vi "Determine Action.vi"(8 "Updated View":i32[](array[numeric]) caption="Updated View (-1 team, 0 empty, 1 enemy)", 9 "Column":i32, 10 "Row":i32, 11 "Great Wall in":refnum<class "Great Wall.lvclass">) -> (1 "Direction":T1, 2 "Action":T2, 3 "Great Wall out":refnum<class "Great Wall.lvclass">)   [LabVIEW 2015, in "Great Wall.lvclass"]
uses:
  Great Wall.lvclass
  DS Square Library/DS Square.lvlib
  Type Defs/Action Enum.ctl
  Type Defs/SB Type Defs.lvlib
  Type Defs/Direction Enum.ctl
  Square/Square.lvclass
  Wall State Enum.ctl
panel:
  # "NW\nN\nNE\nE\nSE\nS\nSW\nW"
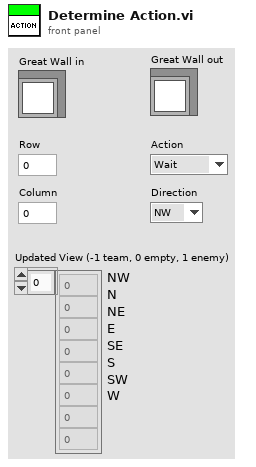
[diagram p1: front panel]
types:
  T1 = typedef "SB Type Defs.lvlib/Direction Enum.ctl" = enum16{"NW", "N", "NE", "E", "SE", "S", "SW", "W"}
  T2 = typedef "SB Type Defs.lvlib/Action Enum.ctl" = enum16{"Wait", "Move", "Attack", "Replicate"}
  T3 = typedef "Great Wall.lvclass/Wall State Enum.ctl" = enum16{"Under Construction", "Hold", "Advance 1", "Advance 2", "Retreat"}
  T4 = typedef "Great Wall.lvclass/Private Data.ctl" = cluster{"wall 1":T5, "wall 2":T5, "start row":i32, "start col":i32, "state update round":i32}
  T5 = typedef "Great Wall.lvclass/Wall State.ctl" = cluster{"state":T3, "direction":T1, "index":i32}
  T6 = typedef "Great Wall.lvclass/Square Mode.ctl" = enum16{"Replicator", "Guard", "Wall"}
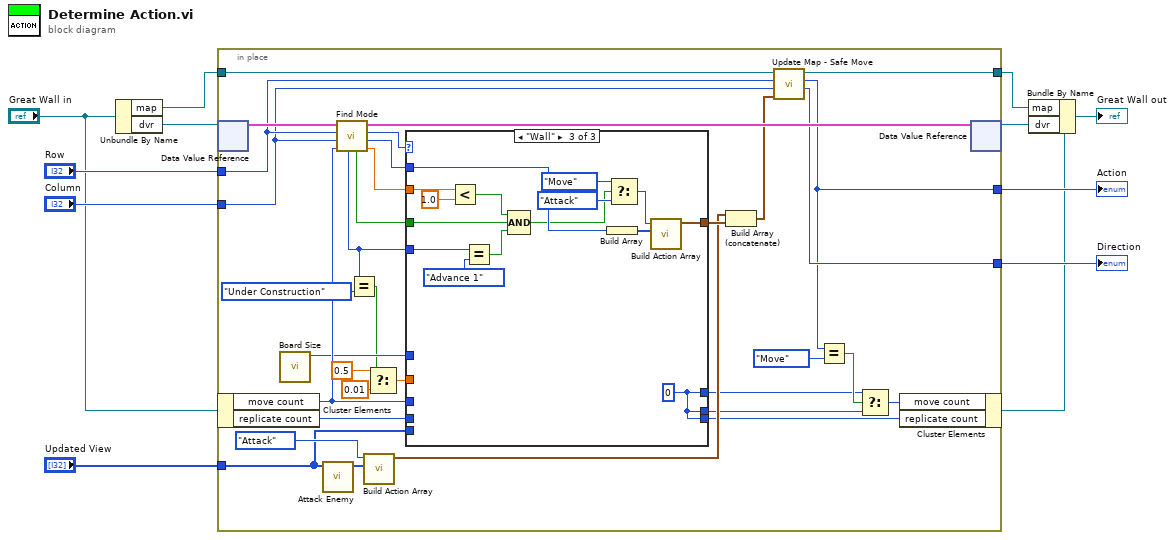
[diagram p0: block diagram]
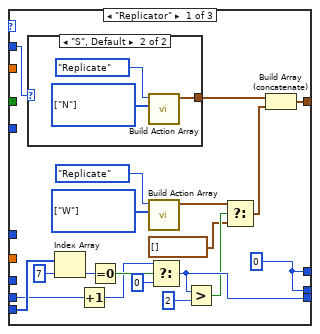
[diagram p2: hidden frame]
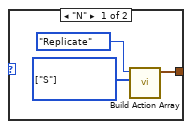
[diagram p3: hidden frame]
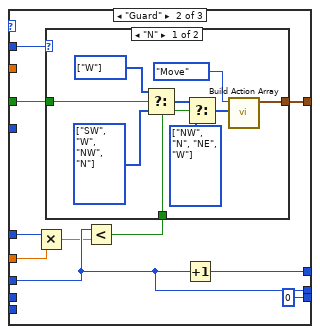
[diagram p4: hidden frame]
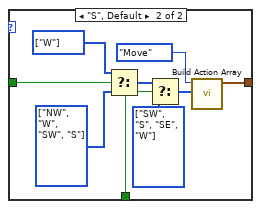
[diagram p5: hidden frame]
diagram:
  n1 = Unbundle By Name("Great Wall in") -> ("map"=w7:refnum<data-value>, "dvr"=w12:refnum<data-value>)
  n2 = in-place {
    in-place-border: "Row" -> [w34]
    in-place-border: "Column" -> [w33]
    in-place-border: w7 -> [w44]
    in-place-border: "Updated View" -> [w21]
    in-place-border: [w43] -> w5
    in-place-border: [w31] -> w4
    in-place-border: [w32] -> w3
    n3 = in-place-dvr #1(w12) -> (w45:T4)  [unwired: 1 out]
    n4 = in-place-cluster #2("Great Wall in") -> ("move count"=w25:i32, "replicate count"=w24:i32)
    n5 = call "Board Size.vi"() -> ("Board Size"=w20:i32)  [unwired: 11 in]
    n6 = call "Attack Enemy.vi"("View in"=w21) -> ("all enemies"=w22:T1[])  [unwired: 8 in, 2 out]
    n7 = call "Find Mode.vi"("move count"=w25, "Column"=w33, "Row"=w34, "private data in"=w45) -> ("distance"=w13:dbl, "nearest wall"=w39:T1, "mode"=w41:T6, "private data out"=w42:T4, "even?"=w35:bool, "wall state"=w19:T3)  [unwired: 2 in]
    n8 = Equal?(x=w19, y=Wall_State_Enum."Under Construction") -> (x = y?=w17:bool)
    n9 = call "Build Action Array.vi"("directions"=w22, "Action"=Action_Enum."Attack") -> ("actions"=w37:cluster{"Action":T2, "Direction":T1}[])  [unwired: 9 in]
    n10 = Select(t=0.5, s=w17, f=0.01) -> (s? t:f=w16:dbl)
    n11 = case shown="\"Wall\"" w41 {
      tunnel: w39 -> [w64 w80 w112]
      tunnel: [w60 w79 w113] -> w38
      tunnel: w25 -> [_ w75 _]
      tunnel: [w63 w78 w105] -> w28
      tunnel: w35 -> [_ w77 w104]
      tunnel: [w63 w75 w105] -> w26
      tunnel: w19 -> [_ _ w110]
      tunnel: w24 -> [w53 _ _]
      tunnel: [w50 0 ("replicate count") w105] -> w23
      tunnel: w21 -> [w57 _ _]
      tunnel: w20 -> [_ w72 _]
      tunnel: w16 -> [_ w71 _]
      tunnel: w13 -> [_ _ w101]
      frame "Replicator" {
        w61 = T1[] [enum."W"] items=["NW", "N", "NE", "E", "SE", "S", "SW", "W"] ("all enemies")
        w63 = 0
        n12 = case shown="\"S\", Default" w64 {
          tunnel: [w65 w68] -> w59
          frame "N" {
            w67 = T1[] [enum."S"] items=["NW", "N", "NE", "E", "SE", "S", "SW", "W"] ("all enemies")
            n13 = call "Build Action Array.vi"("directions"=w67, "Action"=Action_Enum."Replicate") -> ("actions"=w65:cluster{"Action":T2, "Direction":T1}[])  [unwired: 9 in]
          }
          frame "S", Default {
            w70 = T1[] [enum."N"] items=["NW", "N", "NE", "E", "SE", "S", "SW", "W"] ("all enemies")
            n14 = call "Build Action Array.vi"("directions"=w70, "Action"=Action_Enum."Replicate") -> ("actions"=w68:cluster{"Action":T2, "Direction":T1}[])  [unwired: 9 in]
          }
        }
        n15 = Index Array(array=w57, index=7) -> (element=w55:i32)
        n16 = Increment(x=w53) -> (x+1=w52:i32)
        n17 = Equal To 0?(x=w55) -> (x = 0?=w54:bool)
        n18 = call "Build Action Array.vi"("directions"=w61, "Action"=Action_Enum."Replicate") -> ("actions"=w58:cluster{"Action":T2, "Direction":T1}[])  [unwired: 9 in]
        n19 = Select(t=w52, s=w54, f=0) -> (s? t:f=w50:i32)
        n20 = Greater?(x=w50, y=2) -> (0:w48:bool)
        n21 = Select(t=w58, s=w48, f=cluster{"Action":T2, "Direction":T1}[] []) -> (s? t:f=w46:cluster{"Action":T2, "Direction":T1}[])
        n22 = Build Array (concatenate)(w59, w46) -> (w60:cluster{"Action":T2, "Direction":T1}[])
      }
      frame "Guard" {
        n23 = Multiply(x=w72, y=w71) -> (x*y=w73:dbl)
        n24 = Less?(x=w75, y=w73) -> (x < y?=w76:bool)
        n25 = case shown="\"N\"" w80 {
          tunnel: [w88 w97] -> w79
          tunnel: w77 -> [w85 w94]
          tunnel: w76 -> [w81 w90]
          frame "N" {
            w82 = T1[] [enum."NW", enum."N", enum."NE", enum."W"] items=["NW", "N", "NE", "E", "SE", "S", "SW", "W"] ("all enemies")
            w86 = T1[] [enum."W"] items=["NW", "N", "NE", "E", "SE", "S", "SW", "W"] ("all enemies")
            w87 = T1[] [enum."SW", enum."W", enum."NW", enum."N"] items=["NW", "N", "NE", "E", "SE", "S", "SW", "W"] ("all enemies")
            n26 = Select(t=w86, s=w85, f=w87) -> (s? t:f=w84:T1[])
            n27 = Select(t=w84, s=w81, f=w82) -> (s? t:f=w83:T1[])
            n28 = call "Build Action Array.vi"("directions"=w83, "Action"=Action_Enum."Move") -> ("actions"=w88:cluster{"Action":T2, "Direction":T1}[])  [unwired: 9 in]
          }
          frame "S", Default {
            w91 = T1[] [enum."SW", enum."S", enum."SE", enum."W"] items=["NW", "N", "NE", "E", "SE", "S", "SW", "W"] ("all enemies")
            w95 = T1[] [enum."W"] items=["NW", "N", "NE", "E", "SE", "S", "SW", "W"] ("all enemies")
            w96 = T1[] [enum."NW", enum."W", enum."SW", enum."S"] items=["NW", "N", "NE", "E", "SE", "S", "SW", "W"] ("all enemies")
            n29 = Select(t=w95, s=w94, f=w96) -> (s? t:f=w93:T1[])
            n30 = Select(t=w93, s=w90, f=w91) -> (s? t:f=w92:T1[])
            n31 = call "Build Action Array.vi"("directions"=w92, "Action"=Action_Enum."Move") -> ("actions"=w97:cluster{"Action":T2, "Direction":T1}[])  [unwired: 9 in]
          }
        }
        n32 = Increment(x=w75) -> (x+1=w78:i32)
      }
      frame "Wall" {
        w105 = 0
        n33 = Less?(x=w101, y=1.0) -> (x < y?=w99:bool)
        n34 = Equal?(x=w110, y=Wall_State_Enum."Advance 1" ("wall state")) -> (x = y?=w103:bool)
        n35 = Compound Arithmetic op=AND(w99, w104, w103) -> (w102:bool)
        n36 = Build Array(w112) -> (w111:T1[])
        n37 = Select(t=Action_Enum."Move" ("Action"), s=w102, f=Action_Enum."Attack" ("Action")) -> (s? t:f=w108:T2)
        n38 = call "Build Action Array.vi"("directions"=w111, "Action"=w108) -> ("actions"=w113:cluster{"Action":T2, "Direction":T1}[])  [unwired: 9 in]
      }
    }
    n39 = Build Array (concatenate)(w37, w38) -> (w36:cluster{"Action":T2, "Direction":T1}[])
    n40 = call "Update Map - Safe Move.vi"("Action Order"=w36, "Column"=w33, "Row"=w34, "map in"=w44) -> ("Selected Direction"=w32:T1, "Selected Action"=w31:T2, "map out"=w43:refnum<data-value>)  [unwired: 4 in, 1 out]
    n41 = Equal?(x=w31, y=Action_Enum."Move") -> (x = y?=w29:bool)
    n42 = Select(t=w28, s=w29, f=w26) -> (s? t:f=w27:i32)
    n43 = in-place-cluster #2("move count"=w27, "replicate count"=w23) -> (w1:refnum<class "Great Wall.lvclass">)
    n44 = in-place-dvr #1(w42) -> (w10:refnum<data-value>)  [unwired: 1 out]
  }
  "Action" <- w4
  "Direction" <- w3
  n45 = Bundle By Name(cluster=w1, "map"=w5, "dvr"=w10) -> (→"Great Wall out":refnum<class "Great Wall.lvclass">)
